vi "DemoCode.vi"() -> ()   [LabVIEW 2019]
uses:
  <vilib>/Analysis/Matrix/Datatypes/RealMatrix.ctl
  <vilib>/Analysis/Matrix/NI_Matrix.lvlib
panel:
  out "3D Picture 2":refnum<vi>(3d-picture)
  out "A x B":T1=[[1.0, 0.0, 0.0, 0.0], [0.0, 6.123233995736766e-17, 1.0, 0.0], [0.0, -1.0, 6.123233995736766e-17, 0.0], [0.0, 0.0, 0.0, 1.0]] format="%#_2g"
  in  "Joints":T2(array[cluster])=[{"Theta"=0.0, "d"=0.0, "a"=0.0, "alpha (degrees)"=0.0}] {"alpha (degrees)" format="%.2f"; "a" format="%.2f"; "d" scale=0.0..0.5; "Theta" scale=-180.0..180.0}
  in  "Start":T1=[[1.0, 0.0, 0.0, 0.0], [0.0, 1.0, 0.0, 0.0], [0.0, 0.0, 1.0, 0.0], [0.0, 0.0, 0.0, 1.0]]
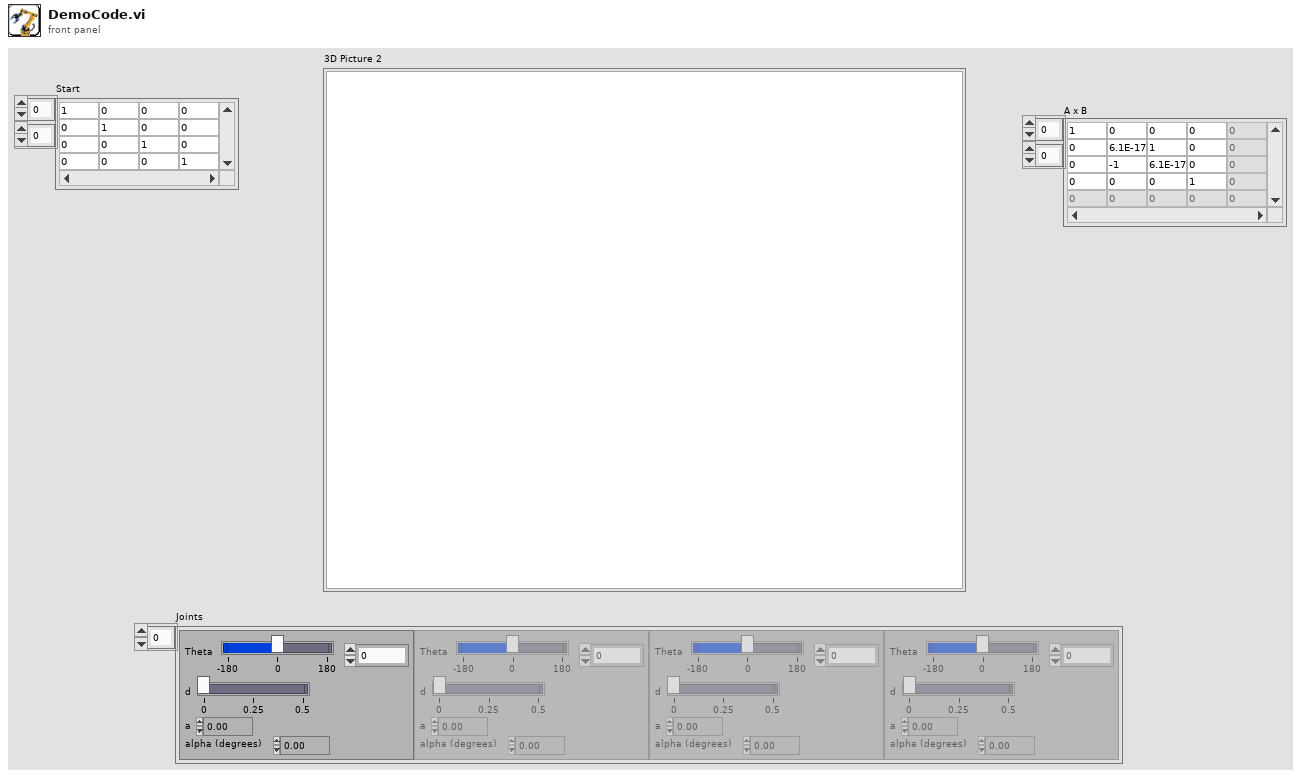
[diagram p1: front panel]
types:
  T1 = typedef "NI_Matrix.lvlib/RealMatrix.ctl" = dbl[][]
  T2 = cluster{"Theta":dbl, "d":dbl, "a":dbl, "alpha (degrees)":dbl}[]
  T3 = cluster{"Line width":sgl, "Line Color":u32, "Axes?":bool}
  T4 = cluster{"Theta (degrees)":dbl, "d":dbl, "a":dbl, "alpha (degrees)":dbl}
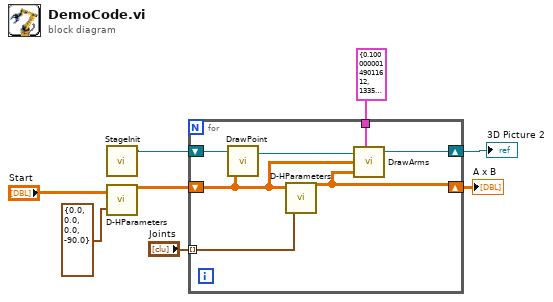
[diagram p0: block diagram]
diagram:
  n1 = call <userlib>:"StageInit.vi"() -> ("Stage out"=w8:refnum<vi>)  [unwired: 4 in, 1 out]
  n2 = call <userlib>:"D-HParameters.vi"("n+1"=T4 {"Theta (degrees)"=0.0, "d"=0.0, "a"=0.0, "alpha (degrees)"=-90.0}, "Start"="Start") -> ("A x B"=w1:T1)  [unwired: 1 in]
  n3 = for {
    shift-right: [w13] -> w4
    shift-left: w1 -> [w9]
    tunnel: "Joints" -> [w15] mode=indexing
    tunnel: T3 {"Line width"=0.1, "Line Color"=13354149, "Axes?"=TRUE} ("Params") -> [w14]
    shift-right: [w12] -> w2
    shift-left: w8 -> [w11]
    n4 = call <userlib>:"DrawPoint.vi"("Start"=w9, "Stage in"=w11) -> ("Stage out"=w10:refnum<vi>)  [unwired: 1 in]
    n5 = call <userlib>:"D-HParameters.vi"("n+1"=w15, "Start"=w9) -> ("A x B"=w13:T1)  [unwired: 1 in]
    n6 = call <userlib>:"DrawArms.vi"("Stage in"=w10, "Params"=w14, "Start"=w9, "End"=w13) -> ("Stage out"=w12:refnum<vi>)  [unwired: 2 in, 1 out]
  }
  "A x B" <- w4
  "3D Picture 2" <- w2
